vi "testDataPass_v1,0_vi2.vi"() -> ()   [LabVIEW 2014]
panel:
  out "arrTF_read":bool[](array[boolean])
  in  "stop":bool
  in  "Read Location":string="dstp://localhost/wave"
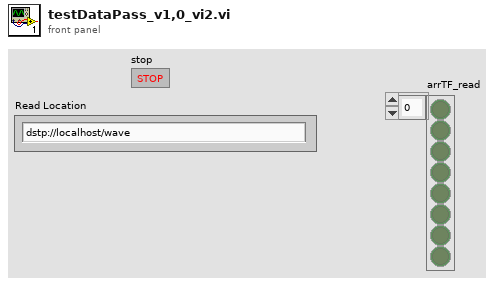
[diagram p1: front panel]
types:
  T1 = enum16{"Read", "Write", "ReadWrite", "BufferedRead", "BufferedReadWrite"}
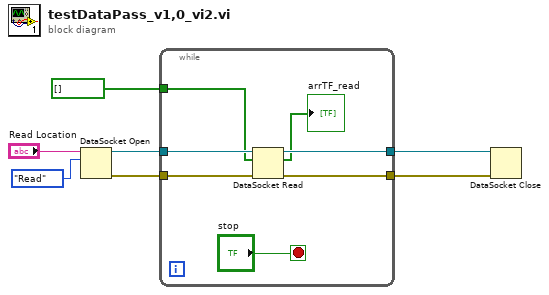
[diagram p0: block diagram]
diagram:
  n1 = DataSocket Open(10:T1."Read" ("mode"), 11:"Read Location") -> (0:w4:errorcluster, 3:w5:refnum<k13>)  [unwired: 2 in]
  n2 = while {
    tunnel: w5 -> [w12]
    tunnel: w4 -> [w13]
    tunnel: [w11] -> w3
    tunnel: [w10] -> w2
    tunnel: bool[] [] ("arrTF_read") -> [w9]
    stop <- "stop" stop-if-true
    n3 = DataSocket Read(8:w13, 10:w9, 11:w12) -> (0:w10:errorcluster, 2:→"arrTF_read":bool[], 3:w11:refnum<k13>)  [unwired: 1 in, 5 out]
  }
  n4 = DataSocket Close(8:w2, 11:w3) -> ()  [unwired: 1 in, 2 out]
